vi "Output on.vi"(8 "error in (no error)":errorcluster, 10 "Output On":bool, 11 "E3631A in":refnum<class "E3631A.lvclass">) -> (0 "error out":errorcluster, 3 "E3631A out":refnum<class "E3631A.lvclass">)   [LabVIEW 2020, in "E3631A.lvclass"]
uses:
  E3631A.lvclass
  C:/Sandbox/Git_Sandbox/WiSpry Test Framework source code (LV20)/WiSpry Test Framework/Instruments/Power Supply/Power Supply.lvclass
  C:/Sandbox/Git_Sandbox/WiSpry Test Framework source code (LV20)/WiSpry Test Framework/Instruments/Instrument.lvclass
  Instrument.lvclass/Instrument.ctl
  Power Supply.lvclass/Power Supply.ctl
  Instrument.lvclass
  Power Supply.lvclass
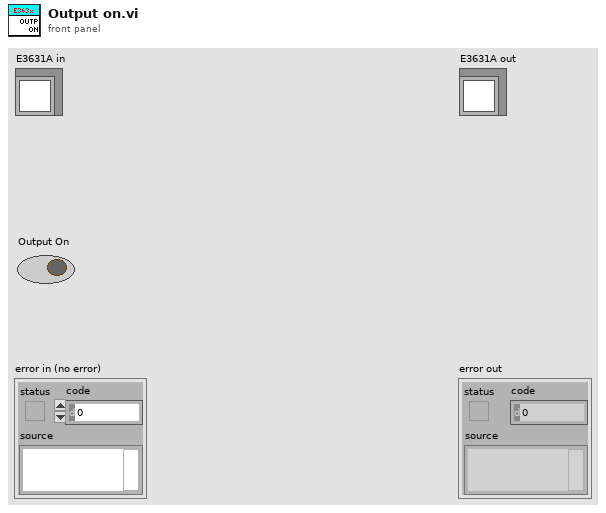
[diagram p1: front panel]
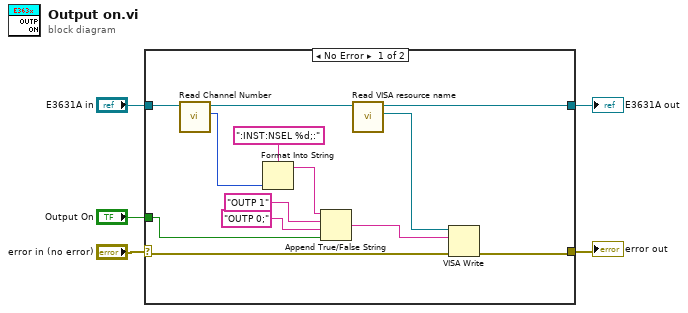
[diagram p0: block diagram]
diagram:
  n1 = case shown="No Error" "error in (no error)" {
    selector: "error in (no error)" -> [w16 w20]
    tunnel: [w17 w20] -> w4
    tunnel: "E3631A in" -> [w8 w19]
    tunnel: [w18 w19] -> w2
    tunnel: "Output On" -> [w10 _]
    frame No Error {
      n2 = call "Read Channel Number.vi"("Power Supply in"=w8) -> ("Channel Number"=w6:u8, "Power Supply out"=w7:refnum<class "E3631A.lvclass">)  [unwired: 9 in]
      n3 = Format Into String(format string=":INST:NSEL %d;:", w6) -> (resulting string=w13:string)  [unwired: 2 in, 1 out]
      n4 = Append True/False String(1:w10, 2:"OUTP 0;" ("false string"), 3:"OUTP 1" ("true string"), 4:w13) -> (0:w9:string)
      n5 = call "Read VISA resource name.vi"("Instrument in"=w7) -> ("VISA resource name"=w15:refnum<visa-resource-name>, "Instrument out"=w18:refnum<class "E3631A.lvclass">)  [unwired: 9 in]
      n6 = VISA Write(VISA resource name=w15, write buffer=w9, error in (no error)=w16) -> (error out=w17:errorcluster)  [unwired: 2 out]
    }
    frame Error {
    }
  }
  "error out" <- w4
  "E3631A out" <- w2
